vi "Write StdWaveformParams.vi"(8 "error in (no error)":errorcluster, 10 "StdWaveformParams":T1={"eWaveform"=0, "dAmplitude"=0.1, "dDcOffset"=0.0, "dFrequency"=1000.0, "dStartPhase"=1000.0, "dSampleRate"=1000.0, "dNumSamples"=1000.0} {"eWaveform" items=["Sine"=0, "Square"=1, "Ramp"=2, "Noise"=3, "DC"=4, "Triangle"=5, "Pulse"=6, "Sinc"=11, "D-Lorentz"=12, "Gaussian"=13, "Expo Fall"=14, "Expo Rise"=15, "Haversine"=16]}, 11 "NISTFGenPluginsBase in":refnum<class "NISTFGenPluginsBase.lvclass">) -> (0 "error out":errorcluster, 3 "NISTFGenPluginsBase out":refnum<class "NISTFGenPluginsBase.lvclass">)   [LabVIEW 2014, in "FGenPlugins.lvlib" / "NISTFGenPluginsBase.lvclass"]
uses:
  NISTFGenPluginsBase.lvclass
  TypeDef/StdWaveformParams.ctl
  NISTFGenPluginsBase.lvclass/NISTFGenPluginsBase.ctl
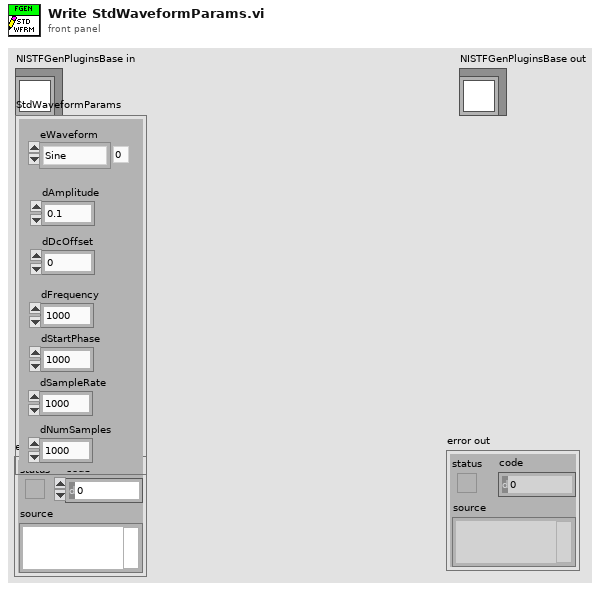
[diagram p1: front panel]
types:
  T1 = typedef "FGenPlugins.lvlib/NISTFGenPluginsBase.lvclass/StdWaveformParams.ctl" = cluster{"eWaveform":u16, "dAmplitude":dbl, "dDcOffset":dbl, "dFrequency":dbl, "dStartPhase":dbl, "dSampleRate":dbl, "dNumSamples":dbl}
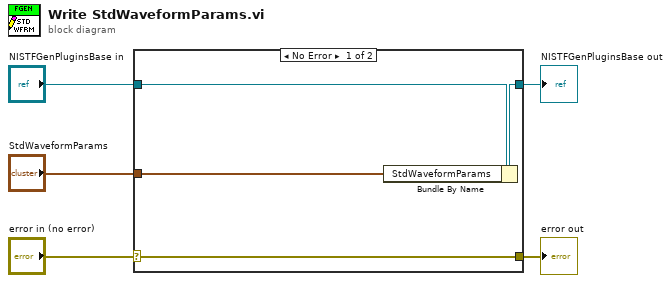
[diagram p0: block diagram]
diagram:
  n1 = case shown="No Error" "error in (no error)" {
    selector: "error in (no error)" -> [w9 w10]
    tunnel: [w9 w10] -> w4
    tunnel: [w7 w11] -> w2
    tunnel: "NISTFGenPluginsBase in" -> [w8 w11]
    tunnel: "StdWaveformParams" -> [w6 _]
    frame No Error {
      n2 = Bundle By Name(cluster=w8, "StdWaveformParams"=w6) -> (w7:refnum<class "NISTFGenPluginsBase.lvclass">)
    }
    frame Error {
    }
  }
  "error out" <- w4
  "NISTFGenPluginsBase out" <- w2
